vi "comm error flags.vi"(1 "Error Flags":u32 format="%.0x") -> (0 "error flags cluster":T1)   [LabVIEW 2017, in "lvserial.lvlib"]
doc: "Decodes the error flags from Comm Status.vi"
uses:
  lvserial.lvlib
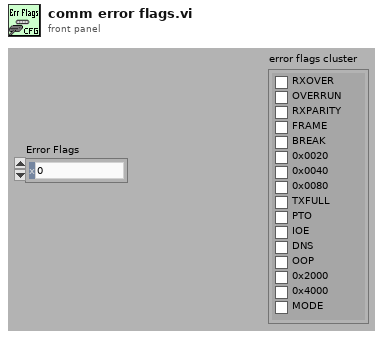
[diagram p1: front panel]
types:
  T1 = cluster{"RXOVER":bool, "OVERRUN":bool, "RXPARITY":bool, "FRAME":bool, "BREAK":bool, "0x0020":bool, "0x0040":bool, "0x0080":bool, "TXFULL":bool, "PTO":bool, "IOE":bool, "DNS":bool, "OOP":bool, "0x2000":bool, "0x4000":bool, "MODE":bool}
  T2 = cluster{"Boolean array[0]":bool, "Boolean array[1]":bool, "Boolean array[2]":bool, "Boolean array[3]":bool, "Boolean array[4]":bool, "Boolean array[5]":bool, "Boolean array[6]":bool, "Boolean array[7]":bool, "Boolean array[8]":bool, "Boolean array[9]":bool, "Boolean array[10]":bool, "Boolean array[11]":bool, "Boolean array[12]":bool, "Boolean array[13]":bool, "Boolean array[14]":bool, "Boolean array[15]":bool}
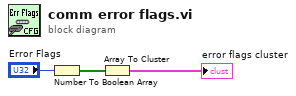
[diagram p0: block diagram]
diagram:
  n1 = Number To Boolean Array(number="Error Flags") -> (Boolean array=w2:bool[])
  n2 = Array To Cluster(array=w2) -> (cluster=→"error flags cluster":T2)
